vi "P612_Ctrl_Index.vi"(5 "OldVal":variant, 11 "NewVal":variant) -> (4 "Control out":refnum<vi>, 8 "P612 out":T1)   [LabVIEW 2014]
uses:
  Type Defs/P612.ctl
panel:
  in  "P612 in":T1
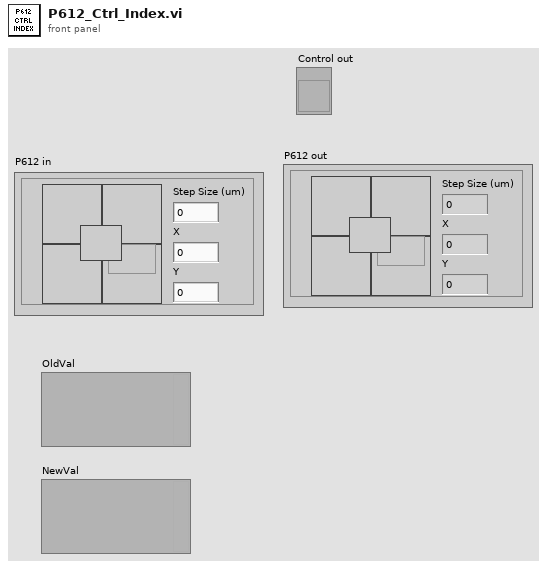
[diagram p1: front panel]
types:
  T1 = typedef "P612.ctl" = cluster{"Home Button":bool, "Up Button":bool, "Left Button":bool, "Down Button":bool, "Right Button":bool, "Step Size (um)":dbl, "X":dbl, "Y":dbl}
  T2 = cluster{"Home Button":bool, "Up Button":bool, "Left Button":bool, "Down Button":bool, "Right Button":bool, "Step Size (um)":bool, "X":bool, "Y":bool}
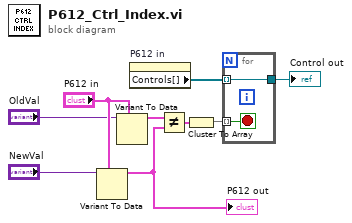
[diagram p0: block diagram]
diagram:
  n1 = Variant To Data(type="P612 in", Variant="NewVal") -> (data=w8:T1)  [unwired: 1 in, 1 out]
  "P612 out" <- w8
  n2 = Variant To Data(type="P612 in", Variant="OldVal") -> (data=w3:T1)  [unwired: 1 in, 1 out]
  n3 = property on="P612 in" class="Clust"() -> ("Controls[]"=w1:refnum<vi>[])  [unwired: 2 in, 2 out]
  n4 = Not Equal?(x=w3, y=w8) -> (x != y?=w7:T2)
  n5 = Cluster To Array(cluster=w7) -> (array=w4:bool[])
  n6 = for {
    tunnel: w4 -> [w10] mode=indexing
    tunnel: w1 -> [w11] mode=indexing
    tunnel: [w11] -> w2
    stop <- w10 stop-if-true
  }
  "Control out" <- w2
